vi "AudioTest.Read Limit File, Output to Plot Item.vi"(8 "error in":errorcluster, 10 "Plot Template":T1={"Order"=0, "Name"="Freq Response", "X"=[], "Y"=[], "X Units"="dB", "Y Units"="Hz", "LimitType"=enum."None", "FailCode"=0, "FailDesc"="", "Ref Data Name"="", "Result Name"="", "0dB Level"=0.0, "Normalized"=FALSE}, 11 "Limit File":path) -> (0 "error out":errorcluster, 2 "UL":T1, 3 "LL":T1)   [LabVIEW 2018]
uses:
  TypeDefs/AudioTest.Result Plot Data.ctl
  Common/Utils/Errors/Error.Error Code List.ctl
  <vilib>/KATE/Files/File Utils.lvlib
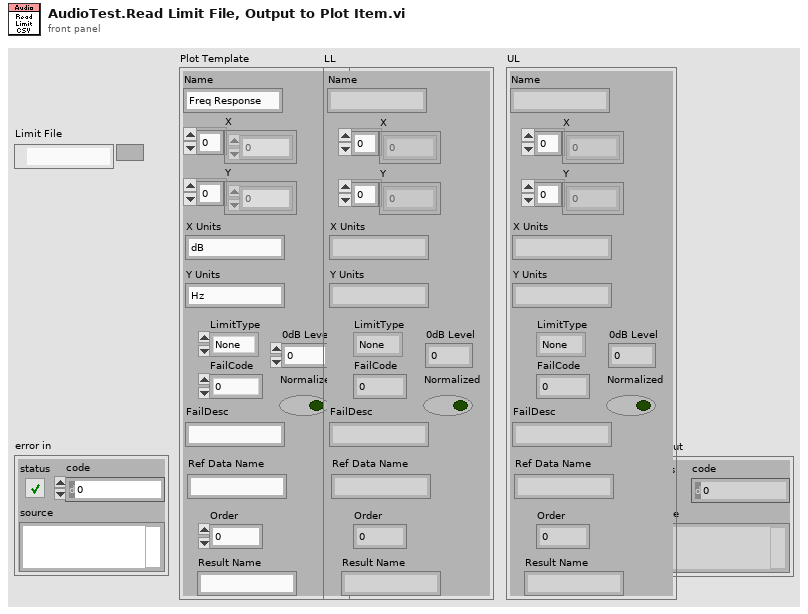
[diagram p1: front panel]
types:
  T1 = typedef "AudioTest.Result Plot Data.ctl" = cluster{"Order":i32, "Name":string, "X":dbl[], "Y":dbl[], "X Units":string, "Y Units":string, "LimitType":enum16{"None", "LL", "UL"}, "FailCode":i32, "FailDesc":string, "Ref Data Name":string, "Result Name":string, "0dB Level":dbl, "Normalized":bool}
  T2 = typedef "Error.Error Code List.ctl" = i32
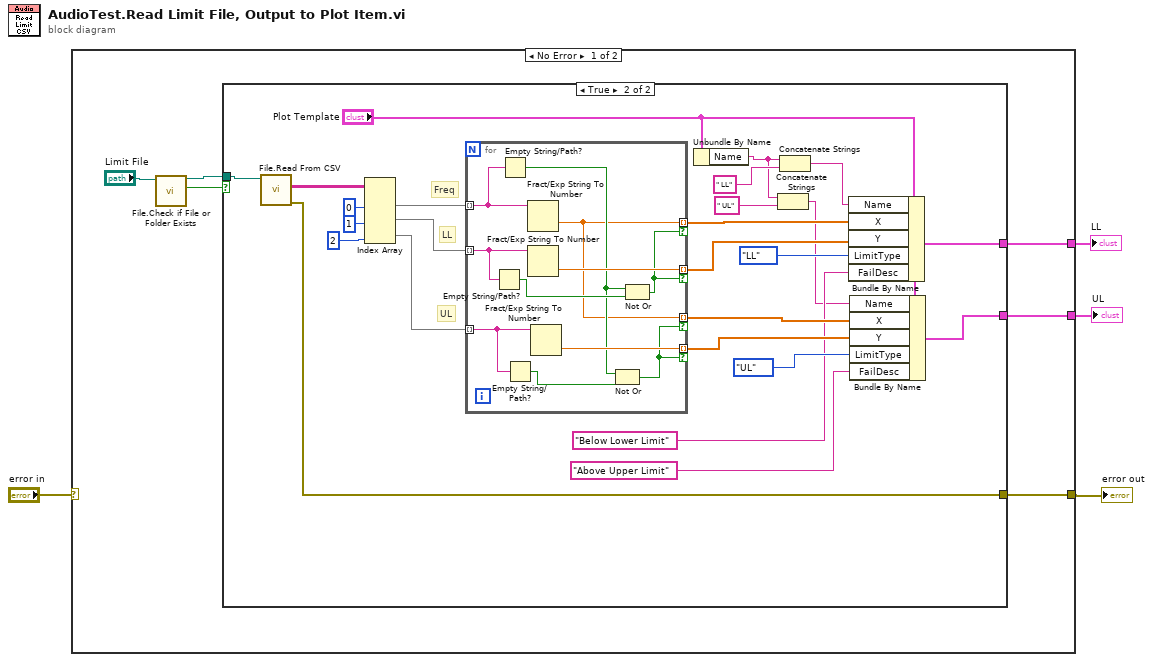
[diagram p0: block diagram]
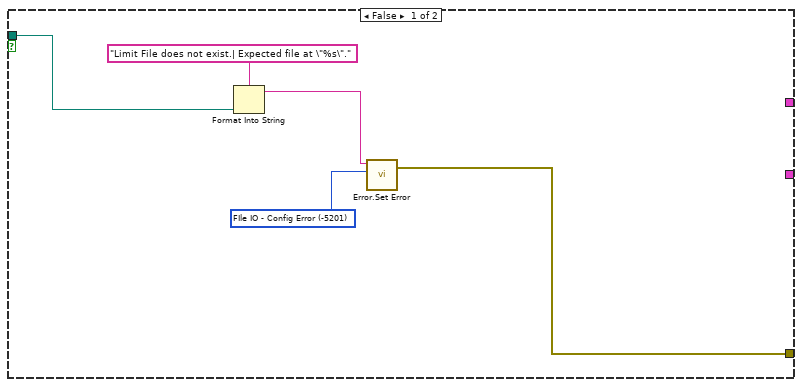
[diagram p2: hidden frame]
diagram:
  n1 = case shown="No Error" "error in" {
    selector: "error in" -> [_ w52]
    tunnel: [w7 w52] -> w3
    tunnel: [w6 _] -> w2
    tunnel: [w5 _] -> w1
    frame No Error {
      n2 = call <vilib>:"File.Check if File or Folder Exists.vi"("Path"="Limit File") -> ("Exists"=w9:bool, "Dup Path"=w8:path)  [unwired: 6 in, 3 out]
      n3 = case shown="True" w9 {
        tunnel: w8 -> [w12 w35]
        tunnel: [w11 w34] -> w7
        tunnel: [_ w29] -> w6
        tunnel: [_ w28] -> w5
        frame False {
          w15 = T2 -5201 items=["No Error"=0, "Abort"=-2, "Misc"=-5000, "Fixture Error"=-5100, "File IO - General"=-5200, "FIle IO - Config Error"=-5201, "Instrument - General"=-5300, "Instrument - Serial Com"=-5301, "Instrument - Camera"=-5302, "Instrument - PS"=-5303, "Instrument - Oscilloscope"=-5304, "Instrument - Function Gen"=-5305, "Instrument - Load"=-5306, "Instrument - Meter"=-5307, "Instrument - Power Control"=-5308, "Instrument - Motion"=-5309, "Instrument - RF"=-5310, "System Exe"=-5400, "Image Processing"=-5500, "Communication"=-5600, "Script - Syntax Error"=-6000, "Script - Invalid Name or Param"=-6100, "Script - Timeout"=-6200, "Invalid Data"=-6300, "FW Update Error"=-6500] ("Std Code")
          n4 = Format Into String(format string="Limit File does not exist.| Expected file at \"%s\".", w12) -> (resulting string=w14:string)  [unwired: 2 in, 1 out]
          n5 = call "Error.Set Error.vi"("Code"=w15, "Desc"=w14) -> ("error out"=w11:errorcluster)  [unwired: 5 in]
        }
        frame True {
          # "UL"
          # "Freq"
          # "LL"
          n6 = call <vilib>:"File.Read From CSV.vi"("File"=w35) -> ("error out"=w34:errorcluster, "Data"=w40:string[][])  [unwired: 8 in, 1 out]
          n7 = Index Array(array=w40, index (col) #1=0 ("disabled index (col)"), index (col) #2=1 ("index (col)"), index (col) #3=2 ("index (col)")) -> (element #1=w37:string[], element #2=w36:string[], element #3=w25:string[])  [unwired: 3 in]
          n8 = for {
            tunnel: w37 -> [w49] mode=indexing
            tunnel: w36 -> [w47] mode=indexing
            tunnel: [w51] -> w32 mode=indexing if=w41
            tunnel: [w43] -> w27 mode=indexing if=w41
            tunnel: [w50] -> w26 mode=indexing if=w42
            tunnel: w25 -> [w48] mode=indexing
            tunnel: [w43] -> w24 mode=indexing if=w42
            n9 = Empty String/Path?(string/path=w47) -> (empty?=w46:bool)
            n10 = Empty String/Path?(string/path=w49) -> (empty?=w44:bool)
            n11 = Empty String/Path?(string/path=w48) -> (empty?=w45:bool)
            n12 = Fract/Exp String To Number(string=w49) -> (number=w43:dbl)  [unwired: 3 in, 1 out]
            n13 = Fract/Exp String To Number(string=w47) -> (number=w51:dbl)  [unwired: 3 in, 1 out]
            n14 = Fract/Exp String To Number(string=w48) -> (number=w50:dbl)  [unwired: 3 in, 1 out]
            n15 = Not Or(1:w45, 2:w44) -> (0:w42:bool)
            n16 = Not Or(1:w46, 2:w44) -> (0:w41:bool)
          }
          n17 = Unbundle By Name("Plot Template") -> ("Name"=w18:string)
          n18 = Concatenate Strings(w18, " UL") -> (w16:string)
          n19 = Concatenate Strings(w18, " LL") -> (w19:string)
          n20 = Bundle By Name(cluster="Plot Template", "Name"=w19, "X"=w27, "Y"=w32, "LimitType"=enum16{"None", "LL", "UL"}."LL", "FailDesc"="Below Lower Limit") -> (w29:T1)
          n21 = Bundle By Name(cluster="Plot Template", "Name"=w16, "X"=w24, "Y"=w26, "LimitType"=enum16{"None", "LL", "UL"}."UL", "FailDesc"="Above Upper Limit") -> (w28:T1)
        }
      }
    }
    frame Error {
    }
  }
  "error out" <- w3
  "LL" <- w2
  "UL" <- w1
